vi "Get Properties.vi"(8 "error in":errorcluster, 10 "AppInst":refnum<vi>, 11 "VI Name":string caption="VI Name (\"\")") -> (0 "error out":errorcluster, 1 "Column Data Type":enum16{"String", "Numeric"}[](array[ring]), 2 "Column Labels":string[](array[string])=["VI Name", "State", "Reentrant", "Reentrancy Type", "FP Behavior", "Code Size", "Data Size", "VI Path"], 3 "Full Name Out":string, 4 "VI Properties":string[](array[string]), 5 "File Name Out":string)   [LabVIEW 2011]
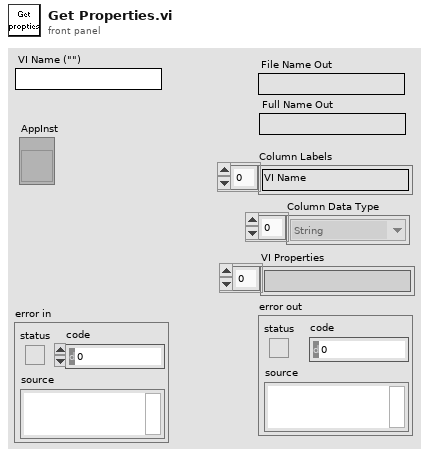
[diagram p1: front panel]
types:
  T1 = enum32{"Bad", "Idle", "Run top level", "Running"}
  T2 = enum16{"Share clones between instances", "Preallocate clone for each instance"}
  T3 = enum32{"Invalid", "Default", "Floating", "Floating/Auto-Hide", "Modal"}
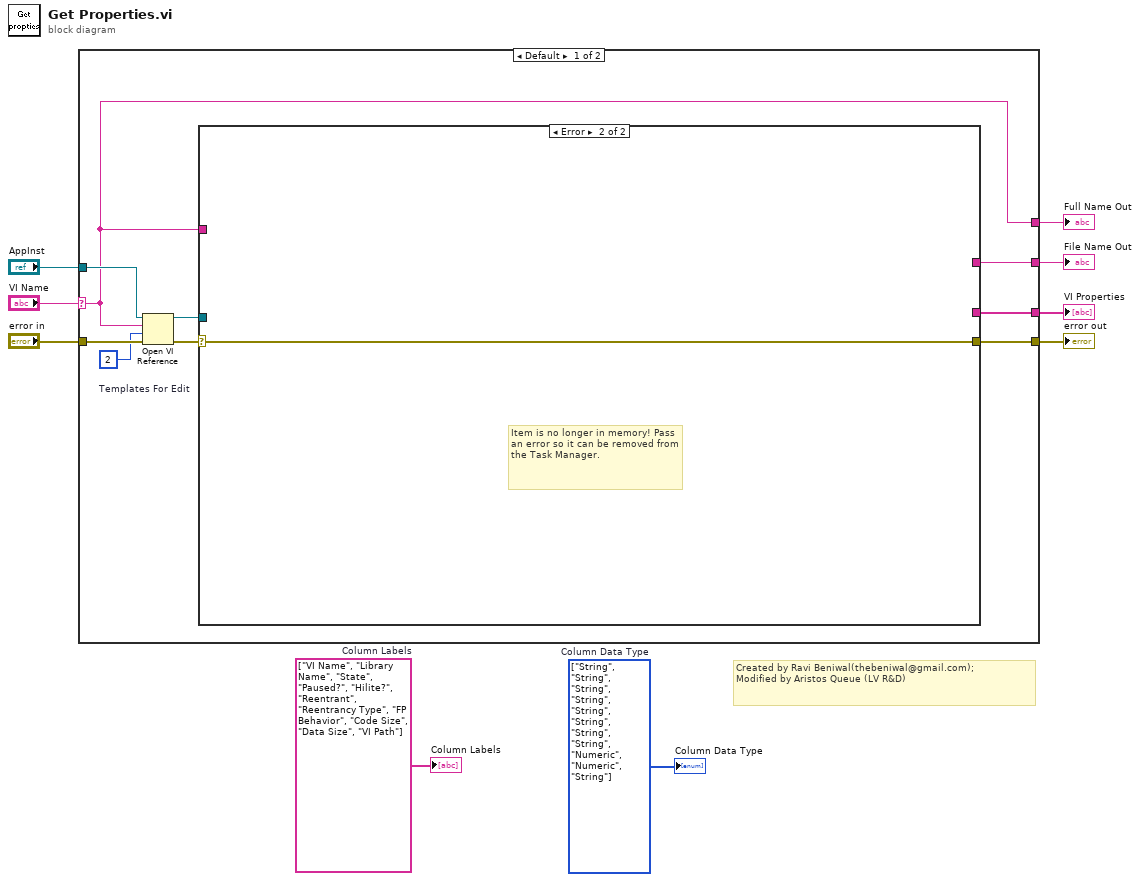
[diagram p0: block diagram]
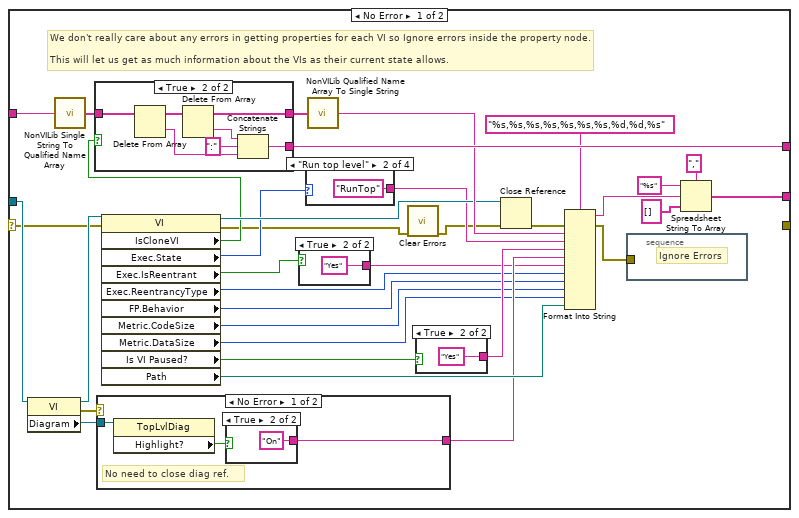
[diagram p2: hidden frame]
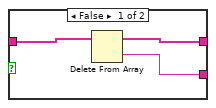
[diagram p3: hidden frame]
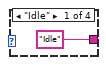
[diagram p5: hidden frame]
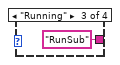
[diagram p6: hidden frame]
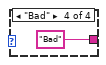
[diagram p7: hidden frame]
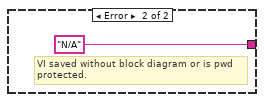
[diagram p9: hidden frame]
diagram:
  w5 = enum16{"String", "Numeric"}[] [enum."String", enum."String", enum."String", enum."String", enum."String", enum."String", enum."String", enum."String", enum."Numeric", enum."Numeric", enum."String"] items=["String", "Numeric"]  # Column Data Type
  w8 = string[] ["VI Name", "Library Name", "State", "Paused?", "Hilite?", "Reentrant", "Reentrancy Type", "FP Behavior", "Code Size", "Data Size", "VI Path"]  # Column Labels
  # "Created by Ravi Beniwal(thebeniwal@gmail.com);\nModified by Aristos Queue (LV R&D)"
  n1 = case shown="Default" "VI Name" {
    selector: "VI Name" -> [w12 w76]
    tunnel: [w18 _] -> w9
    tunnel: "error in" -> [w17 w75]
    tunnel: [w12 w76] -> w6
    tunnel: [w14 _] -> w4
    tunnel: "AppInst" -> [w13 _]
    tunnel: [w10 w75] -> w1
    frame Default {
      w15 = 2  # Templates For Edit
      n2 = Open VI Reference(application reference (local)=w13, vi path=w12, options=w15, error in (no error)=w17) -> (vi reference=w16:refnum<vi>, error out=w11:errorcluster)  [unwired: 2 out]
      n3 = case shown="Error" w11 {
        selector: w11 -> [w19 w74]
        tunnel: [w52 _] -> w18
        tunnel: w16 -> [w51 _]
        tunnel: [w50 _] -> w14
        tunnel: w12 -> [w49 _]
        tunnel: [_ w74] -> w10
        frame No Error {
          # "We don't really care about any errors in getting properties for each VI so Ignore errors inside the property node.\n\nThis will let us get as much information about the VIs as their current state allows."
          n4 = property class="VI"(reference=w51) -> (reference out=w35:refnum<vi>, error out=w36:errorcluster, "Diagram"=w34:refnum<vi>)  [unwired: 1 in]
          n5 = call "NonVILib Single String To Qualified Name Array.vi"("Fully Qualified String"=w49) -> ("Fully Qualified Array"=w48:string[])
          n6 = case shown="No Error" w36 {
            tunnel: [w68 "N/A"] -> w30
            tunnel: w34 -> [w70 _]
            frame No Error {
              # "No need to close diag ref."
              n7 = property class="TopLvlDiag"(reference=w70) -> ("Highlight?"=w69:bool)  [unwired: 1 in, 2 out]
              n8 = case shown="True" w69 {
                tunnel: [_ "On"] -> w68
                frame False {
                }
                frame True {
                }
              }
            }
            frame Error {
              # "VI saved without block diagram or is pwd protected."
            }
          }
          n9 = property class="VI"(reference=w35, error in=w19) -> (reference out=w45:refnum<vi>, error out=w20:errorcluster, "IsCloneVI"=w22:bool, "Exec.State"=w33:T1, "Exec.IsReentrant"=w25:bool, "Exec.ReentrancyType"=w26:T2, "FP.Behavior"=w27:T3, "Metric.CodeSize"=w28:u32, "Metric.DataSize"=w29:u32, "Is VI Paused?"=w37:bool, "Path"=w38:path)
          n10 = case shown="True" w22 {
            tunnel: w48 -> [w55 w62]
            tunnel: [w54 w56] -> w50
            tunnel: [w53 w60] -> w47
            frame False {
              n11 = Delete From Array(array=w55) -> (deleted portion=w54:string, array with subset deleted=w53:string[])  [unwired: 2 in]
            }
            frame True {
              n12 = Delete From Array(array=w62) -> (deleted portion=w58:string, array with subset deleted=w61:string[])  [unwired: 2 in]
              n13 = Delete From Array(array=w61) -> (deleted portion=w59:string, array with subset deleted=w60:string[])  [unwired: 2 in]
              n14 = Concatenate Strings(w59, ":" ("element"), w58) -> (w56:string)
            }
          }
          n15 = case shown="True" w25 {
            tunnel: [_ "Yes"] -> w24
            frame False {
            }
            frame True {
            }
          }
          n16 = case shown="\"Run top level\"" w33 {
            tunnel: ["Idle" "RunTop" "RunSub" "Bad"] -> w32
            frame "Idle" {
            }
            frame "Run top level" {
            }
            frame "Running" {
            }
            frame "Bad" {
            }
          }
          n17 = call "NonVILib Qualified Name Array To Single String.vi"("Fully Qualified Array"=w47) -> ("Fully Qualified String"=w46:string)
          n18 = call <vilib>:"Clear Errors.vi"("error in (no error)"=w20) -> ("error out"=w21:errorcluster)  [unwired: 6 in]
          n19 = case shown="True" w37 {
            tunnel: [_ "Yes"] -> w31
            frame False {
            }
            frame True {
            }
          }
          n20 = Close Reference(reference=w45, error in (no error)=w21) -> (error out=w42:errorcluster)
          n21 = Format Into String(format string="%s,%s,%s,%s,%s,%s,%s,%d,%d,%s", error in=w42, w46, w32, w31, w30, w24, w26, w27, w28, w29, w38) -> (resulting string=w39:string, error out=w23:errorcluster)  [unwired: 1 in]
          n22 = stacked-sequence {
            tunnel: w23 -> [_]
            frame #0 {
              # "Ignore Errors"
            }
          }
          n23 = Spreadsheet String To Array(delimiter (Tab)=",", format string="%s", spreadsheet string=w39, array type (2D Dbl)=string[] [] ("appended array")) -> (array=w52:string[])
        }
        frame Error {
          # "Item is no longer in memory! Pass an error so it can be removed from the Task Manager."
        }
      }
    }
    frame "" {
      # "Addin this blank case let's us use this VI for getting the Col headers. \nIt is just easier to manage the column headers and getting their values in one VI."
    }
  }
  "error out" <- w1
  "VI Properties" <- w9
  "Full Name Out" <- w6
  "File Name Out" <- w4
  "Column Labels" <- w8
  "Column Data Type" <- w5
